vi "CRYGet Graph Window Information.vi"(0 "pGraph VI In":refnum<vi>) -> (1 "Queue Name Out":string, 2 "Cursor Ref Out":refnum<vi>, 3 "Graph Number Out":i32, 4 "pGraph VI Out":refnum<vi>, 6 "Garph Title Out":string, 8 "Graph Type Out":string, 10 "Graph Control Ref Out":variant, 12 "CursorShow Out":bool, 13 "Legend Splitter Position":dbl, 14 "LegendShow Out":bool, 15 "Legend Ref Out":refnum<vi>)   [LabVIEW 2013]
panel:
  out "bResult":bool=TRUE
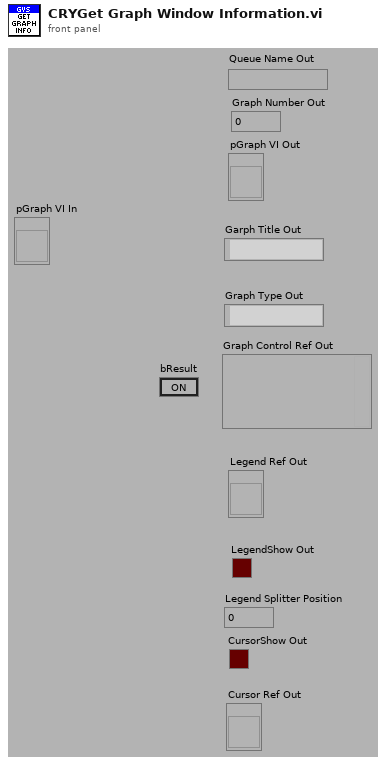
[diagram p1: front panel]
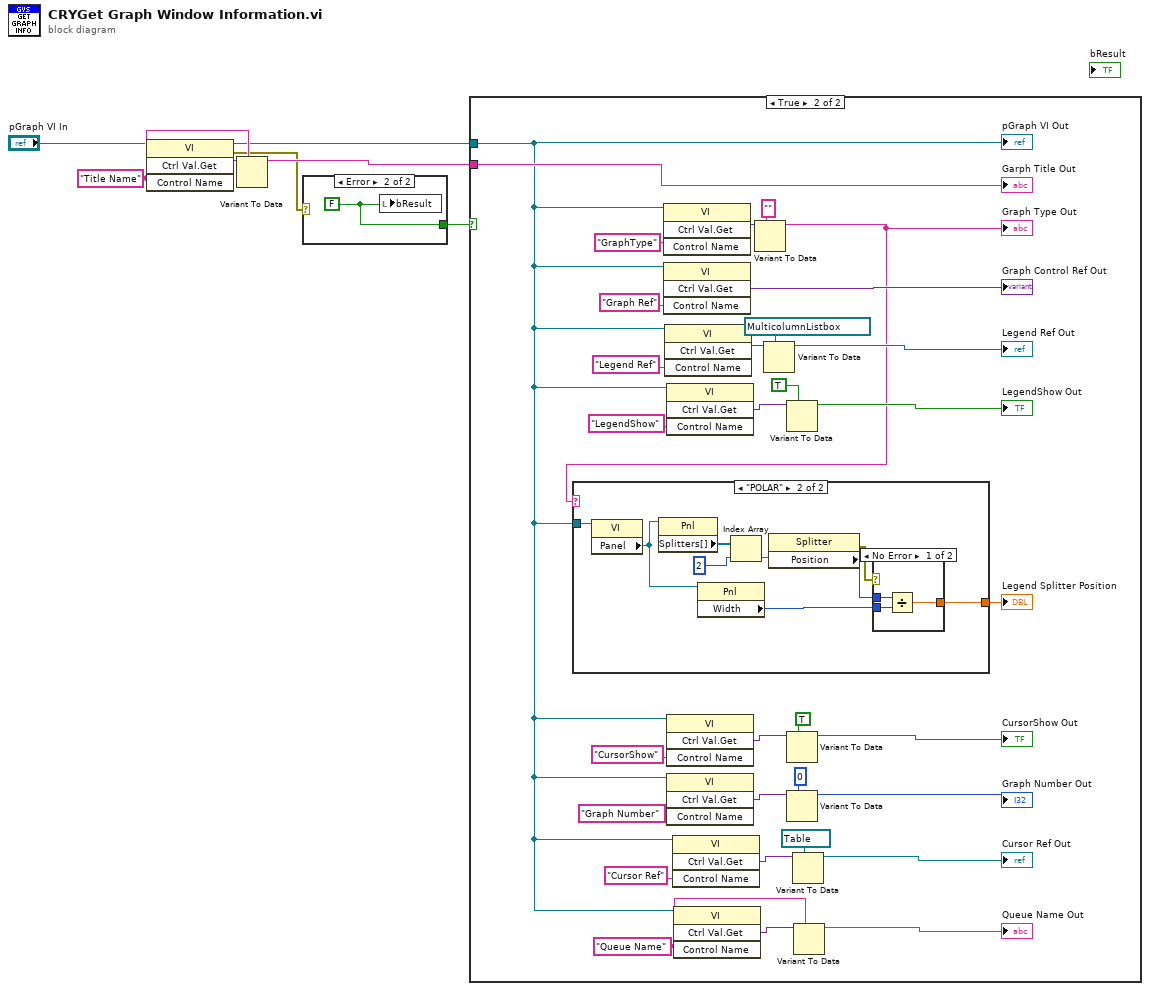
[diagram p0: block diagram]
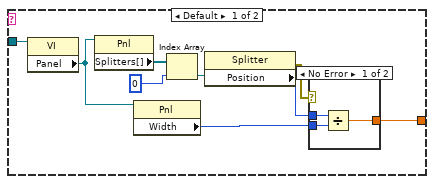
[diagram p3: hidden frame]
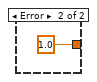
[diagram p4: hidden frame]
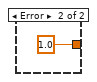
[diagram p5: hidden frame]
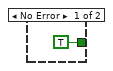
[diagram p6: hidden frame]
diagram:
  w7 = "Title Name" ("Control Name")
  n1 = invoke class="VI" method="Ctrl Val.Get"(reference="pGraph VI In", "Control Name"=w7) -> (reference out=w2:refnum<vi>, error out=w4:errorcluster, "Get Control Value Variant"=w6:variant)  [unwired: 2 in, 1 out]
  n2 = Variant To Data(type=w7, Variant=w6) -> (data=w5:string)  [unwired: 1 in, 1 out]
  n3 = case shown="Error" w4 {
    tunnel: [TRUE w9] -> w1
    frame No Error {
    }
    frame Error {
      w9 = FALSE
      n4 = local write "bResult"(w9) -> ()
    }
  }
  n5 = case shown="True" w1 {
    tunnel: w5 -> [_ w37]
    tunnel: w2 -> [_ w12]
    frame False {
    }
    frame True {
      w14 = "Queue Name" ("Control Name")
      n6 = invoke class="VI" method="Ctrl Val.Get"(reference=w12, "Control Name"="GraphType") -> ("Get Control Value Variant"=w40:variant)  [unwired: 2 in, 3 out]
      n7 = invoke class="VI" method="Ctrl Val.Get"(reference=w12, "Control Name"="Graph Ref") -> ("Get Control Value Variant"=→"Graph Control Ref Out":variant)  [unwired: 2 in, 3 out]
      n8 = invoke class="VI" method="Ctrl Val.Get"(reference=w12, "Control Name"="Legend Ref") -> ("Get Control Value Variant"=w30:variant)  [unwired: 2 in, 3 out]
      n9 = invoke class="VI" method="Ctrl Val.Get"(reference=w12, "Control Name"="LegendShow") -> ("Get Control Value Variant"=w35:variant)  [unwired: 2 in, 3 out]
      n10 = invoke class="VI" method="Ctrl Val.Get"(reference=w12, "Control Name"="CursorShow") -> ("Get Control Value Variant"=w27:variant)  [unwired: 2 in, 3 out]
      n11 = invoke class="VI" method="Ctrl Val.Get"(reference=w12, "Control Name"="Graph Number") -> ("Get Control Value Variant"=w23:variant)  [unwired: 2 in, 3 out]
      n12 = invoke class="VI" method="Ctrl Val.Get"(reference=w12, "Control Name"="Cursor Ref") -> ("Get Control Value Variant"=w20:variant)  [unwired: 2 in, 3 out]
      n13 = invoke class="VI" method="Ctrl Val.Get"(reference=w12, "Control Name"=w14) -> ("Get Control Value Variant"=w15:variant)  [unwired: 2 in, 3 out]
      n14 = Variant To Data(type="", Variant=w40) -> (data=w11:string)  [unwired: 1 in, 1 out]
      "Graph Type Out" <- w11
      n15 = case shown="\"POLAR\"" w11 {
        tunnel: [w49 w63] -> w32
        tunnel: w12 -> [w42 w56]
        frame Default {
          n16 = property class="VI"(reference=w42) -> ("Panel"=w50:refnum<vi>)  [unwired: 1 in, 2 out]
          n17 = property class="Pnl"(reference=w50) -> ("Splitters[]"=w48:refnum<vi>[])  [unwired: 1 in, 2 out]
          n18 = property class="Pnl"(reference=w50) -> ("Width"=w45:u32)  [unwired: 1 in, 2 out]
          n19 = Index Array(array=w48, index=0) -> (element=w46:refnum<vi>)
          n20 = property class="Splitter"(reference=w46) -> (error out=w43:errorcluster, "Position"=w44:i32)  [unwired: 1 in, 1 out]
          n21 = case shown="No Error" w43 {
            tunnel: [w53 1.0] -> w49
            tunnel: w45 -> [w52 _]
            tunnel: w44 -> [w51 _]
            frame No Error {
              n22 = Divide(x=w51, y=w52) -> (x/y=w53:dbl)
            }
            frame Error {
            }
          }
        }
        frame "POLAR" {
          n23 = property class="VI"(reference=w56) -> ("Panel"=w55:refnum<vi>)  [unwired: 1 in, 2 out]
          n24 = property class="Pnl"(reference=w55) -> ("Splitters[]"=w62:refnum<vi>[])  [unwired: 1 in, 2 out]
          n25 = property class="Pnl"(reference=w55) -> ("Width"=w59:u32)  [unwired: 1 in, 2 out]
          n26 = Index Array(array=w62, index=2) -> (element=w60:refnum<vi>)
          n27 = property class="Splitter"(reference=w60) -> (error out=w57:errorcluster, "Position"=w58:i32)  [unwired: 1 in, 1 out]
          n28 = case shown="No Error" w57 {
            tunnel: [w66 1.0] -> w63
            tunnel: w59 -> [w65 _]
            tunnel: w58 -> [w64 _]
            frame No Error {
              n29 = Divide(x=w64, y=w65) -> (x/y=w66:dbl)
            }
            frame Error {
            }
          }
        }
      }
      "Legend Splitter Position" <- w32
      n30 = Variant To Data(type=refnum<vi> refnum ("GMListbox"), Variant=w30) -> (data=→"Legend Ref Out":refnum<vi>)  [unwired: 1 in, 1 out]
      n31 = Variant To Data(type=TRUE, Variant=w35) -> (data=→"LegendShow Out":bool)  [unwired: 1 in, 1 out]
      n32 = Variant To Data(type=TRUE, Variant=w27) -> (data=→"CursorShow Out":bool)  [unwired: 1 in, 1 out]
      n33 = Variant To Data(type=0 ("Graph Number"), Variant=w23) -> (data=→"Graph Number Out":i32)  [unwired: 1 in, 1 out]
      n34 = Variant To Data(type=refnum<vi> refnum ("GMListbox"), Variant=w20) -> (data=→"Cursor Ref Out":refnum<vi>)  [unwired: 1 in, 1 out]
      n35 = Variant To Data(type=w14, Variant=w15) -> (data=→"Queue Name Out":string)  [unwired: 1 in, 1 out]
      "pGraph VI Out" <- w12
      "Garph Title Out" <- w37
    }
  }
